vi "Reconnect.vi"(8 "error in (no error)":errorcluster, 11 "Serial Stream in":refnum<class "Serial Stream.lvclass">) -> (0 "error out":errorcluster, 3 "Serial Stream out":refnum<class "Serial Stream.lvclass">)   [LabVIEW 2020, in "Stream-Serial.lvlib" / "Serial Stream.lvclass"]
uses:
  Serial Stream.lvclass
  Serial Stream.lvclass/Serial Stream.ctl
  Client Command.ctl
  Stream-Serial.lvlib
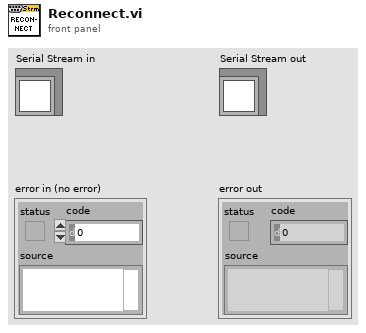
[diagram p1: front panel]
types:
  T1 = typedef "Stream-Serial.lvlib/Client Command.ctl" = enum16{"Connect", "Close", "Shutdown", "Reconnect"}
  T2 = typedef "Stream-Serial.lvlib/Serial Stream.lvclass/Ref Data.ctl" = cluster{"Command Queue":T3}
  T3 = typedef "Stream-Serial.lvlib/Command Queue.ctl" = refnum<queue>
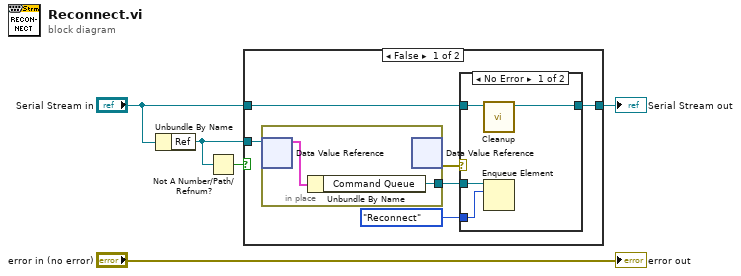
[diagram p0: block diagram]
diagram:
  n1 = Unbundle By Name("Serial Stream in") -> ("Ref"=w4:refnum<data-value>)
  n2 = Not A Number/Path/Refnum?(number/path/refnum=w4) -> (NaN/Path/Refnum?=w3:bool)
  n3 = case shown="False" w3 {
    tunnel: w4 -> [w11 _]
    tunnel: "Serial Stream in" -> [w9 w19]
    tunnel: [w6 w19] -> w1
    frame False {
      n4 = in-place {
        in-place-border: [w17] -> w8
        n5 = in-place-dvr #1(w11) -> (w18:T2)  [unwired: 1 out]
        n6 = Unbundle By Name(w18) -> ("Command Queue"=w17:T3)
        n7 = in-place-dvr #1() -> (w10:errorcluster)  [unwired: 1 in, 1 out]
      }
      n8 = case shown="No Error" w10 {
        tunnel: w9 -> [w13 w16]
        tunnel: w8 -> [w15 _]
        tunnel: Client_Command."Reconnect" ("Command") -> [w14 _]
        tunnel: [w12 w16] -> w6
        frame No Error {
          n9 = call "Cleanup.vi"("Serial Stream in"=w13) -> ("Serial Stream out"=w12:refnum<class "Serial Stream.lvclass">)  [unwired: 9 in, 1 out]
          n10 = Enqueue Element(queue=w15, element=w14) -> ()  [unwired: 2 in, 3 out]
        }
        frame Error {
        }
      }
    }
    frame True {
    }
  }
  "Serial Stream out" <- w1
  "error out" <- "error in (no error)"
